vi "Agilent 34405 Read Single.vi"() -> ()   [LabVIEW 2020]
doc: "This example shows how to configure a measurement and take a single reading."
uses:
  <instrlib>/Agilent 34405/Agilent 34405.lvlib
panel:
  out "Instrument Name":string
  in  "stop":bool
  in  "Function (0: DC Volts)":i32(ring) items=["DC Volts", "AC Volts", "DC Current", "AC Current", "2-Wire Resistance", "Frequency", "Temperature", "Capacitance", "Continuity", "Diode", "4-Wire Resistance", "2nd DC Volts", "2nd AC Volts", "2nd DC Current", "2nd AC Current", "2nd Frequency"]
  in  "Manual Range (1)":dbl=1.0
  in  "Manual Resolution (5.5 Digits)":dbl(ring)=5.5 items=["3.5"=3.5, "4.5"=4.5, "5.5"=5.5]
  in  "Enable Auto Range (T:Enable)":bool=TRUE
  out "Measurement":dbl
  in  "VISA resource name":refnum<visa-resource-name>
  # "(c) 2009 - 2015 National Instruments Corporation.  ALL RIGHTS RESERVED."
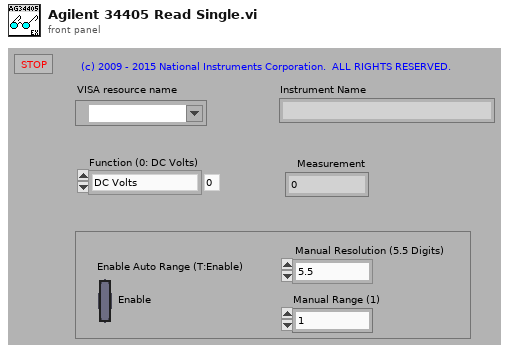
[diagram p1: front panel]
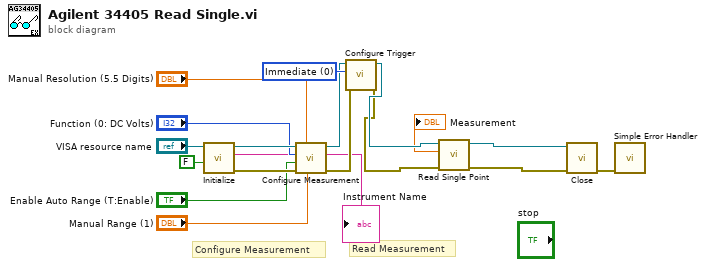
[diagram p0: block diagram]
diagram:
  w8 = 0 items=["Immediate", "Software (Bus)"] ("Trigger Source (0: Immediate)")
  # "Read Measurement"
  # "Configure Measurement"
  n1 = call <instrlib>:"Initialize.vi"("Reset (True)"=FALSE, "VISA resource name"="VISA resource name") -> ("error out"=w15:errorcluster, "Instrument Name"=→"Instrument Name":string, "VISA resource name out"=w16:refnum<visa-resource-name>)  [unwired: 2 in, 5 out]
  n2 = call <instrlib>:"Configure Measurement.vi"("Manual Range (1)"="Manual Range (1)", "Manual Resolution (5.5 Digits)"="Manual Resolution (5.5 Digits)", "error in (no error)"=w15, "Enable Auto Range (T:Enable)"="Enable Auto Range (T:Enable)", "Function (0: DC Volts)"="Function (0: DC Volts)", "VISA resource name"=w16) -> ("error out"=w6:errorcluster, "VISA resource name out"=w7:refnum<visa-resource-name>)  [unwired: 4 out]
  n3 = call <instrlib>:"Configure Trigger.vi"("error in (no error)"=w6, "Trigger Source (0: Immediate)"=w8, "VISA resource name"=w7) -> ("error out"=w4:errorcluster, "VISA resource name out"=w5:refnum<visa-resource-name>)  [unwired: 7 in]
  n4 = call <instrlib>:"Read Single Point.vi"("error in (no error)"=w4, "VISA resource name"=w5) -> ("error out"=w14:errorcluster, "Measurement"=→"Measurement":dbl, "VISA resource name out"=w13:refnum<visa-resource-name>)  [unwired: 7 out]
  n5 = call <instrlib>:"Close.vi"("error in (no error)"=w14, "VISA resource name"=w13) -> ("error out"=w18:errorcluster)  [unwired: 9 out]
  n6 = call <vilib>:"Simple Error Handler.vi"("error in (no error)"=w18) -> ()  [unwired: 1 in, 8 out]
